vi "Continuous Serial Write and Read.vi"() -> ()   [LabVIEW 2021]
doc: "This example performs writes and reads on a serial port, as directed by the user. You can press the Write and Read buttons, and change the Read Count, while the example is running.\n\nThe parameters set for the serial port must match the parameters of the connected instrument or device. In this example, the Read Count parameter specifies the number of bytes that the serial port reads. If there were more bytes at the port than the specified number, those bytes would not be read. If there were less bytes at the port than the specified number, you would receive a timeout error.\n\nThis example expands upon the flow control options for XON and XOFF, allowing the user to choose those control characters. Also, the user can enable or disable a termination character. Some devices require a termination character in order to identify the end of command strings. Some devices send a termination character to signify the end of data to be read. This example shows how you can end the Read operation once a termination character is detected in the buffer and/or append a termination character at the end of the Write data."
uses:
  <vilib>/Instr/_visa.llb/VISA Configure Serial Port (Instr).vi
panel:
  in  "Termination Character":u8=10 format="%.0x"
  in  "End Write on Termination Character?":bool=TRUE
  in  "Stop":bool
  in  "Command":string="CAB-2558"
  in  "Read Count":u32=1000
  out "Response":string
  in  "Write":bool
  in  "Read":bool
  in  "End Read on Termination Character?":bool=TRUE
  in  "VISA resource name":refnum<visa-resource-name>="COM1"
  # "Overview: Demonstrates the use of the VISA functions to write commands to and read responses from a serial instrument continuously in a loop.\nRequirements: NI-VISA Driver\nInstructions:\n1. Run the VI.\n2. Specify a Command and click the Write button.\n3. Read a Response by clicking the Read button.\n4. Click Stop to stop the VI."
  # "0xA is equivalent to a '\\n' character, which is a line feed."
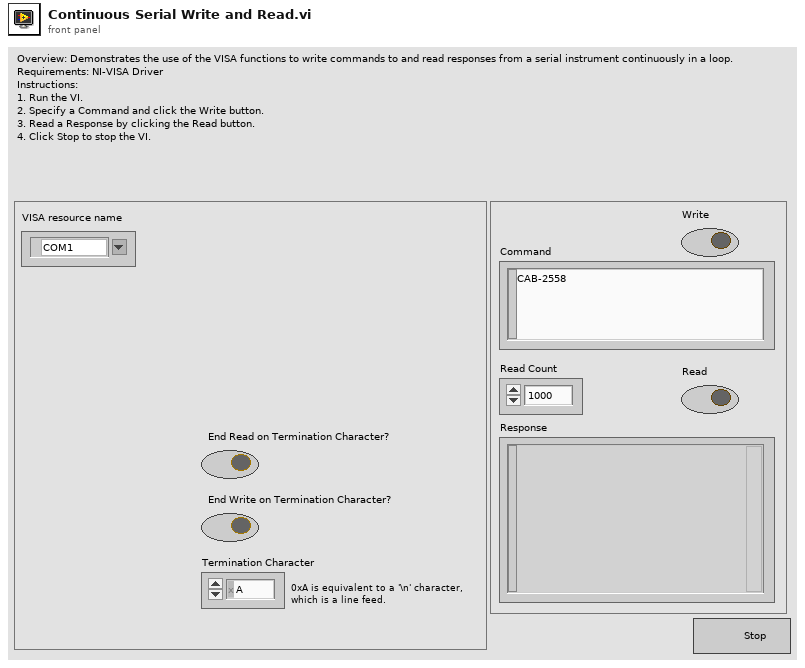
[diagram p1: front panel]
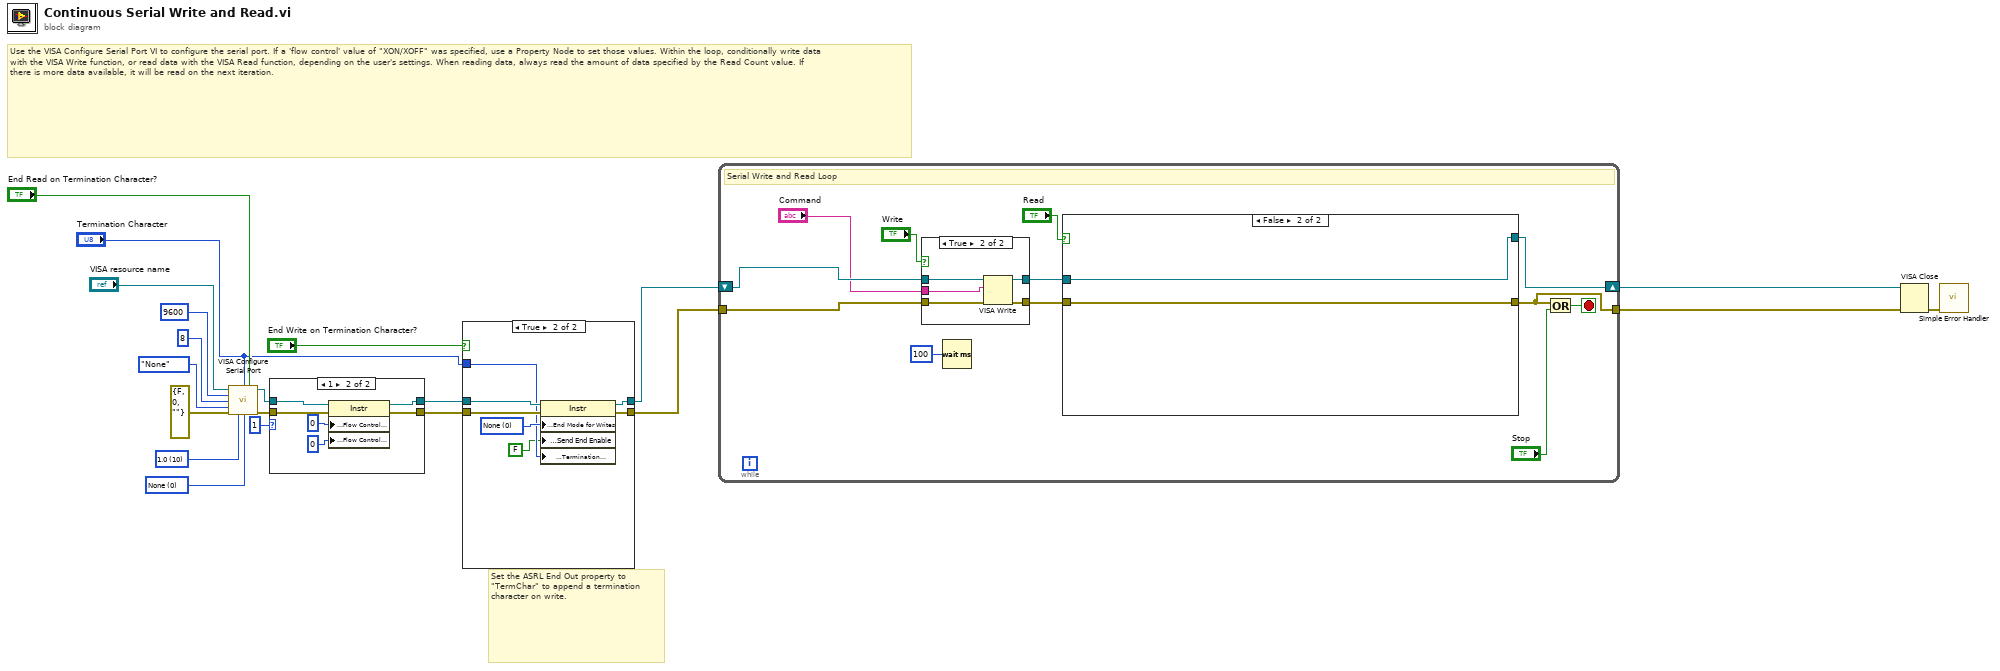
[diagram p0: block diagram]
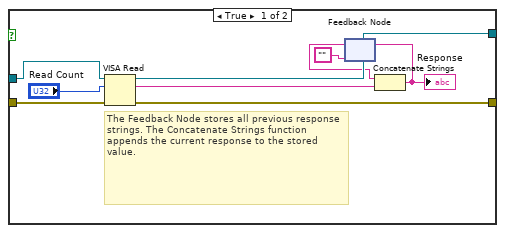
[diagram p5: hidden frame]
diagram:
  w2 = u16 0 items=["None", "XON/XOFF", "RTS/CTS", "XON/XOFF & RTS/CTS", "DTR/DSR", "XON/XOFF & DTR/DSR"] ("flow control (0:none)")
  w3 = u16 10 items=["1.0"=10, "1.5"=15, "2.0"=20] ("stop bits (10: 1 bit)")
  # "Set the ASRL End Out property to \"TermChar\" to append a termination character on write."
  # "Use the VISA Configure Serial Port VI to configure the serial port. If a 'flow control' value of \"XON/XOFF\" was specified, use a Property Node to set those values. Within the loop, conditionally write data with the VISA Write function, or read data with the VISA Read function, depending on the user's settings. When reading data, always read the amount of data specified by the Read Count value. If there is more data available, it will be read on the next iteration."
  n1 = call-poly "VISA Configure Serial Port"("VISA resource name"="VISA resource name", "termination char\n(0xA = '\\n' = LF)"="Termination Character", "Enable Termination\nChar (T)"="End Read on Termination Character?", "baud rate (9600)"=u32 9600, "data bits (8)"=u16 8, "parity (0:none)"=enum16{"None", "Odd", "Even", "Mark", "Space"}."None", "error in (no error)"=errorcluster {"status"=FALSE, "code"=0, "source"=""}, "stop bits (10: 1 bit)"=w3, "flow control (0:none)"=w2) -> ("VISA resource name out"=w18:refnum<visa-resource-name>, "error out"=w19:errorcluster)  [unwired: 1 in, 4 out]
  n2 = case shown="1" u16 1 ("flow control") {
    tunnel: [w21 w28] -> w13
    tunnel: [w22 w27] -> w11
    tunnel: w19 -> [w21 w26]
    tunnel: w18 -> [w22 w25]
    frame Default {
    }
    frame 1 {
      n3 = property class="Instr"(reference=w25, error in=w26, "Serial Settings:Flow Control XON Character"=u8 0, "Serial Settings:Flow Control XOFF Character"=u8 0) -> (reference out=w27:refnum<visa-resource-name>, error out=w28:errorcluster)
    }
  }
  n4 = case shown="True" "End Write on Termination Character?" {
    tunnel: w11 -> [w29 w37]
    tunnel: w13 -> [w30 w36]
    tunnel: [w29 w35] -> w10
    tunnel: [w30 w34] -> w12
    tunnel: "Termination Character" -> [_ w32]
    frame False {
    }
    frame True {
      w33 = u16 0 items=["None", "LastBit", "TermChar", "Break"] ("Serial Settings:Serial End Mode for Writes")
      n5 = property class="Instr"(reference=w37, error in=w36, "Serial Settings:End Mode for Writes"=w33, "Message Based Settings:Send End Enable"=FALSE, "Message Based Settings:Termination Character"=w32) -> (reference out=w35:refnum<visa-resource-name>, error out=w34:errorcluster)
    }
  }
  n6 = while {
    shift-right: [w49] -> w14
    shift-left: w10 -> [w48]
    tunnel: w12 -> [w47]
    tunnel: [w41] -> w15
    stop <- w42 stop-if-true
    # "Serial Write and Read Loop"
    n7 = case shown="True" "Write" {
      tunnel: w48 -> [w51 w56]
      tunnel: w47 -> [w50 w55]
      tunnel: [w51 w54] -> w46
      tunnel: [w50 w53] -> w45
      tunnel: "Command" -> [_ w52]
      frame False {
      }
      frame True {
        n8 = VISA Write(VISA resource name=w56, write buffer=w52, error in (no error)=w55) -> (VISA resource name out=w54:refnum<visa-resource-name>, error out=w53:errorcluster)  [unwired: 1 out]
      }
    }
    n9 = Wait (ms)(milliseconds to wait=u32 100) -> ()  [unwired: 1 out]
    n10 = case shown="False" "Read" {
      tunnel: [w63 w67] -> w49
      tunnel: w46 -> [w65 w67]
      tunnel: [w61 w66] -> w41
      tunnel: w45 -> [w64 w66]
      frame True {
        # "The Feedback Node stores all previous response strings. The Concatenate Strings function appends the current response to the stored value."
        n11 = VISA Read(VISA resource name=w65, byte count="Read Count", error in (no error)=w64) -> (VISA resource name out=w63:refnum<visa-resource-name>, read buffer=w60:string, error out=w61:errorcluster)  [unwired: 1 out]
        n12 = feedback #1("") -> (w59:string)
        n13 = Concatenate Strings(w59, w60) -> (w58:string)
        "Response" <- w58
        n14 = feedback-in #1(w58) -> ()
      }
      frame False {
      }
    }
    n15 = Or(x=w41, y="Stop") -> (x .or. y?=w42:bool)
  }
  n16 = VISA Close(VISA resource name=w14, error in (no error)=w15) -> (error out=w16:errorcluster)
  n17 = call <vilib>:"Simple Error Handler.vi"("error in (no error)"=w16) -> ()  [unwired: 1 in, 8 out]
